vi "SaveKeithleyData.vi"(8 "error in (no error)":errorcluster, 9 "Voltage average":dbl, 11 "Refnum in":refnum<k34>) -> (0 "error out":errorcluster, 3 "Refnum out":refnum<k34>)   [LabVIEW 2017]
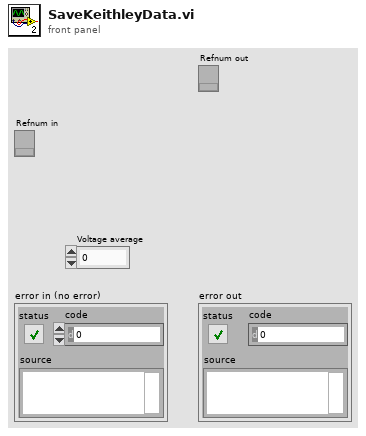
[diagram p1: front panel]
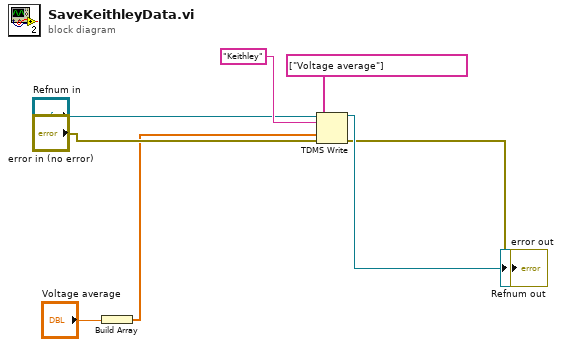
[diagram p0: block diagram]
diagram:
  n1 = Build Array("Voltage average") -> (w1:dbl[])
  n2 = TDMS Write(0:"Refnum in", 5:"Keithley", 7:string[] ["Voltage average"] ("channel name(s) in (Untitled)"), 9:w1, 11:"error in (no error)") -> (4:→"Refnum out":refnum<k34>, 15:→"error out":errorcluster)  [unwired: 1 in, 2 out]
